vi "email debug.vi"() -> ()   [LabVIEW 2019]
uses:
  <vilib>/smtpClient/Set Message Text.vi
  <vilib>/smtpClient/LabVIEWSMTPClient.lvlib
panel:
  out "error out 2":errorcluster
  out "error out":errorcluster
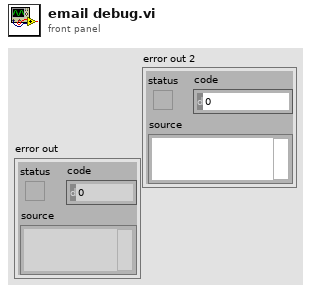
[diagram p1: front panel]
types:
  T1 = typedef "LabVIEWSMTPClient.lvlib/SmtpClientHandle.ctl" = refnum<k1>
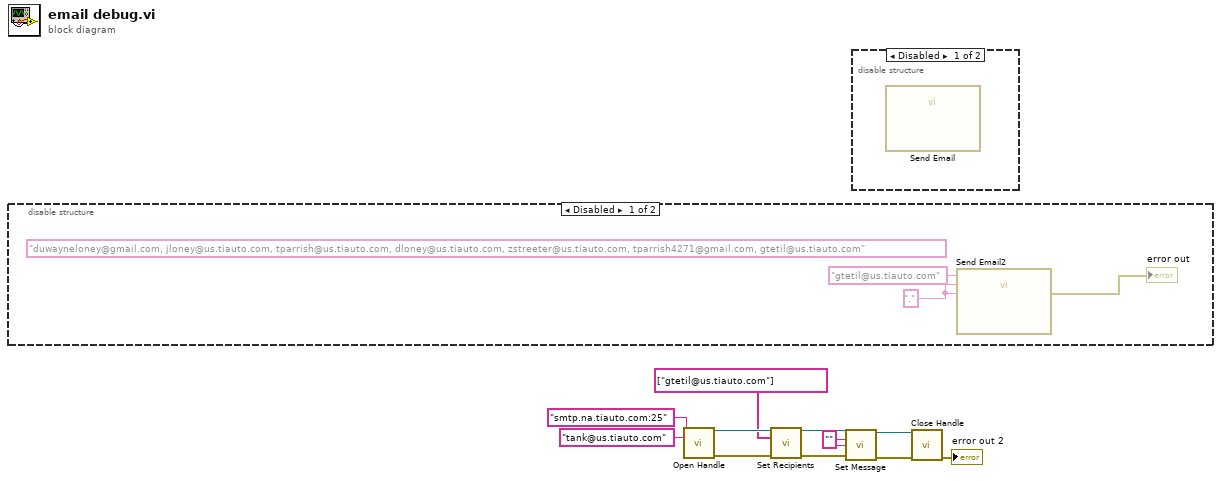
[diagram p0: block diagram]
diagram:
  w1 = "" ("subject")
  n1 = disable-structure shown="Disabled" {
    frame Disabled {
      w12 = "." ("Subject")
      (unwired) "duwayneloney@gmail.com, jloney@us.tiauto.com, tparrish@us.tiauto.com, dloney@us.tiauto.com, zstreeter@us.tiauto.com, tparrish4271@gmail.com, gtetil@us.tiauto.com" ("Recipients")
      n2 = call "Send Email2"("Message"=w12, "Subject"=w12, "Recipients"="gtetil@us.tiauto.com") -> ("error out"=→"error out":errorcluster)  [unwired: 8 in]
    }
    frame Enabled {
    }
  }
  n3 = call <vilib>:"Open Handle.vi"("server address"="smtp.na.tiauto.com:25", "from"="tank@us.tiauto.com") -> ("handle out"=w9:T1, "error out"=w8:errorcluster)  [unwired: 12 in]
  n4 = call <vilib>:"Set Recipients.vi"("handle in"=w9, "to"=string[] ["gtetil@us.tiauto.com"], "error in (no error)"=w8) -> ("handle out"=w6:T1, "error out"=w5:errorcluster)  [unwired: 11 in]
  n5 = call-poly <vilib>:"Set Message.vi"("handle in"=w6, "subject"=w1, "plain text message"=w1, "error in (no error)"=w5) -> ("handle out"=w4:T1, "error out"=w3:errorcluster)  [unwired: 10 in]
  n6 = disable-structure shown="Disabled" {
    frame Disabled {
      n7 = call "Send Email"() -> ()  [unwired: 11 in, 1 out]
    }
    frame Enabled {
    }
  }
  n8 = call <vilib>:"Close Handle.vi"("handle in"=w4, "error in (no error)"=w3) -> ("error out"=→"error out 2":errorcluster)  [unwired: 12 in, 1 out]
